vi "SaveReportPath.vi"() -> ()   [LabVIEW 2013]
doc: "View current datapath and select new."
uses:
  Controls/Enum Save Action Events.ctl
  Globals/DataPathGlobalVariable.vi
  main.lvlib
panel:
  in  "Default":bool
  out "ReportString (transparent)":string caption="Nuværende Mappe"
  in  "ReportCancelBtn":bool
  in  "ReportSaveBtn":bool
  in  "ReportPathCtrl":path caption="Vælg ny mappe"
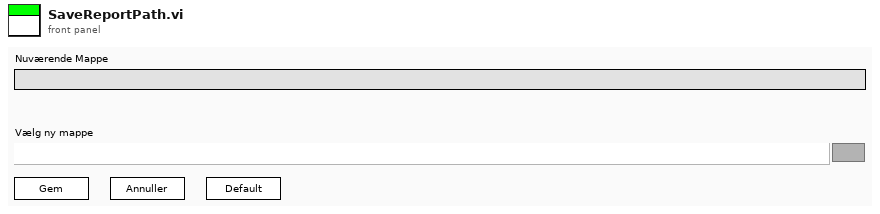
[diagram p1: front panel]
types:
  T1 = typedef "main.lvlib/Enum Save Action Events.ctl" = enum16{"LoadReportPath", "SaveReportPath", "Load Graph Path", "Save Graph Path", "LoadDataPath", "SaveDataPath", "Load Template Path", "Save Template Path", "Load PressureFactor", "Save PressureFactor", "Init", "Load Listbox", "Save Listbox", "LoadHospInfo", "SaveHospInfo", "Load DICOM Activation", "Save DICOM Activation", "LoadDICOMInfoWL", "SaveDICOMInfoWL", "LoadDICOMInfoPACS", "SaveDICOMInfoPACS", "Load ArmCalcMethod", "Save ArmCalcMethod", "LoadItemTags", "SaveItemTags", "LoadDICOMEncoding", "SaveDICOMEncoding", "LoadJournalType", "SaveJournalType", "LoadAcqFilterType", "SaveAcqFilterType", "Load Sequence", "Save Sequence", "Load Acquisition Mode", "Save Acquisition Mode", "Load General Settings", "Save General Settings", "Load Language", "Save Language", "Load Dicom Tags", "Save Dicom Tags", "Load BT Serial", "Save BT Serial", "Load BT License", "Save BT License"}
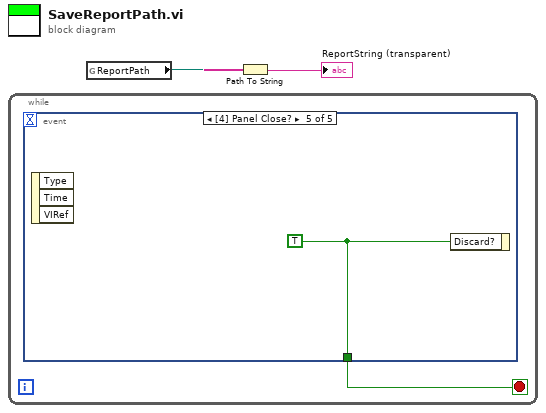
[diagram p0: block diagram]
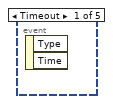
[diagram p2: hidden frame]
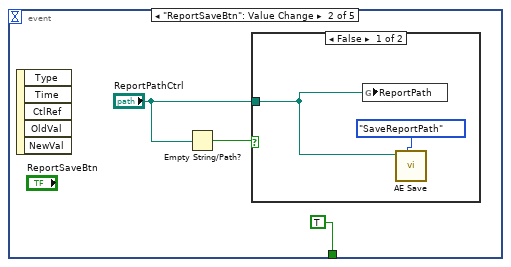
[diagram p3: hidden frame]
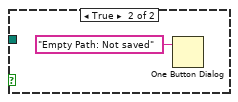
[diagram p4: hidden frame]
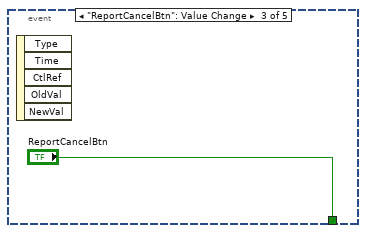
[diagram p5: hidden frame]
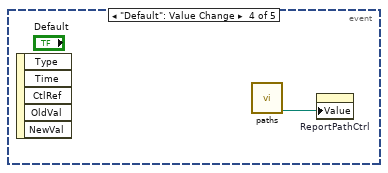
[diagram p6: hidden frame]
diagram:
  n1 = while {
    stop <- w3 stop-if-true
    n2 = event shown="[4] Panel Close?" {
      selector: _ -> [_ _ _ _ _]
      dyn-events: _ -> [_ _ _ _ _]
      timeout: _ -> [_ _ _ _ _]
      tunnel: [_ TRUE "ReportCancelBtn" _ w12] -> w3
      event Timeout {
        n3 = event-data() -> ()  [unwired: 1 in, 2 out]
      }
      event "ReportSaveBtn": Value Change {
        n4 = event-data() -> ()  [unwired: 1 in, 5 out]
        n5 = Empty String/Path?(string/path="ReportPathCtrl") -> (empty?=w4:bool)
        n6 = case shown="False" w4 {
          tunnel: "ReportPathCtrl" -> [w7 _]
          frame False {
            n7 = global write "DataPathGlobalVariable.vi" "ReportPath"(w7) -> ()
            n8 = call "AE Save.vi"("Variant In"=w7, "Action"=Enum_Save_Action_Events."SaveReportPath") -> ()  [unwired: 7 in, 2 out]
          }
          frame True {
            n9 = One Button Dialog(message="Empty Path: Not saved") -> ()  [unwired: 1 in, 1 out]
          }
        }
      }
      event "ReportCancelBtn": Value Change {
        n10 = event-data() -> ()  [unwired: 1 in, 5 out]
      }
      event "Default": Value Change {
        n11 = event-data() -> ()  [unwired: 1 in, 5 out]
        n12 = call "paths.vi"() -> ("Journal Folder"=w11:path)  [unwired: 8 in, 3 out]
        n13 = property on="ReportPathCtrl" class="Path"("Value"=w11) -> ()  [unwired: 2 in, 2 out]
      }
      event Panel Close? {
        w12 = TRUE ("Discard?")
        n14 = event-data() -> ()  [unwired: 1 in, 3 out]
        n15 = event-data("Discard?"=w12) -> ()  [unwired: 1 in, 1 out]
      }
    }
  }
  n16 = global read "DataPathGlobalVariable.vi" "ReportPath"() -> (w1:path)
  n17 = Path To String(path=w1) -> (string=→"ReportString (transparent)":string)
